vi "OntStatus&Info.vi"(8 "error in":errorcluster caption="错误输入（无错误）", 10 "XML document":string="<?xml version=\"1.0\" encoding=\"utf-8\"?>\n<string xmlns=\"http://CIG_WebService/\"><DOC><Row><CIG_SN>FHTXF4112271</CIG_SN><SSID>ChinaNet-Wrgr</SSID><WAP2>7khcpaes</WAP2><WLP>enguz</WLP><ONT_ID>A013CB-48334A013CB3AC294</ONT_ID><provinceID>HG261GS;unipon_patch_5116_Anhui_CTC_20150609_1645</provinceID><Lot>ZH1509290</Lot><PCBA_Code>13U-00032-21</PCBA_Code><MAC1>A013CB3AC294</MAC1><MAC2>A013CB3AC298</MAC2><Major>NA</Major><Minor>NA</Minor><OEM_SN>FHTTCB3AC294</OEM_SN><BOSA_Code>071-85100-00</BOSA_Code><Hwver>NA</Hwver><MCU>NA</MCU><LoadVer>Anhui20150722.rar/U6</LoadVer><Customer_PN>GPON</Customer_PN></Row></DOC></string>\n\n" caption="XML文档", 11 "XPath expression":string="DOC/Row" caption="XPath表达式") -> (0 "error out":errorcluster caption="错误输出", 3 "OntStatus&Info":string[][](array[string]))   [LabVIEW 2012]
uses:
  <vilib>/xml/Load XML String.vi
  <vilib>/xml/Close Reference(Node).vi
  <vilib>/xml/NI_XML.lvlib
  <resource>/objmgr/DOMUserDefRef.rc
panel:
  out "子字符串":string
  in  "偏移量(0)":i32=39
  out "parse errors":string caption="解析出错"
  out "结果字符串":string
  out "数组":string[](array[string])
  out "match found?":bool caption="找到匹配？"
  out "Result XML":string caption="结果XML"
  # "<?xml version=\"1.0\" encoding=\"utf-8\"?>\n<string xmlns=\"http://CIG_WebService/\">\n<DOC><Row><CIG_SN>081690290863</CIG_SN><CheckResult/><Message/><DuplicatedacQty/><SSID/><WAP2>16a0168b</WAP2><WLP/><ONT_ID/><provinceID/><Lot>ZH1610017</Lot><PCBA_Code>15K-00007-21</PCBA_Code><MAC1/><MAC2/><Major>0090</Major><Minor>23</Minor><OEM_SN>081690290863</OEM_SN><FSAN_SN/><BOSA_Code>071-85200-00</BOSA_Code><Hwver>02</Hwver><MCU>NA</MCU><LoadVer>NA</LoadVer><MFG_Date>2016-10-12</MFG_Date><OEM_PCBA_PN/><SSID1_ID/><SSID2_ID/><SSID2_PWD/><WLanMac1/><WLanMac2/><Customer_PN/><LaserSN/><RFPI/><RFPOWER/><DECT_TYPE/><ServiceTag/><Super_Code>15K-90004</Super_Code><IsHuaWei>N</IsHuaWei><BosaQty>1</BosaQty><ONTIP/></Row></DOC></string>"
  # "<?xml version=\"1.0\" encoding=\"utf-8\"?>\n<string xmlns=\"http://CIG_WebService/\"><?xml version=\"1.0\"?>\n<ROOT>\n<HEAD>\n<RC>SFMS_CE_A1</RC>\n<RCNAME>工装计数</RCNAME>\n<APP_ID>{{2F986A52-32F6-C090-5250-B3035315C7E7}}</APP_ID>\n<AUTH_TOKEN>5K@AANDC@HI_QJbQ\\UT^]b_^uhglpppvl|ll</AUTH_TOKEN>\n<RETURNTYPE></RETURNTYPE>\n<TIMESTAMP>2017-08-16 09:57:13</TIMESTAMP>\n<STATUS>1</STATUS>\n<REMARK></REMARK>\n<LGUID>38407521-9ABA-460F-B7E3-BE3CBE1E5FF6</LGUID>\n<SENDTYPE></SENDTYPE>\n<SENDFROM>MES</SENDFROM>\n</HEAD>\n<SFMS_CE_A1>\n<VIN>AL000131-02</VIN>\n<STATUS>Pop</STATUS>\n<ERRORMSG>AL000131-02还有20次到使用次数，请及时保养！</ERRORMSG>\n</SFMS_CE_A1>\n</ROOT></string>"
  # "<?xml version=\"1.0\" encoding=\"utf-8\"?>\n<string xmlns=\"http://CIG_WebService/\"><?xml version=\"1.0\"?>\n<ROOT>\n<HEAD>\n<RC>MSSF_MTO_A2</RC>\n<RCNAME>工单ATE测试软件信息</RCNAME>\n<APP_ID>{5C128BE7-0FB2-3CCB-4A41-821E960FCCF1}</APP_ID>\n<AUTH_TOKEN>8H8;COTH@E][MJRdfgT]la`^kgh~tsollllz</AUTH_TOKEN>\n<RETURNTYPE></RETURNTYPE>\n<TIMESTAMP>2017-03-15 14:01:22</TIMESTAMP>\n<STATUS>1</STATUS>\n<REMARK>PRD_10000004</REMARK>\n<LGUID>5C128BE7-0FB2-3CCB-4A41-821E960FCCF1</LGUID>\n<SENDTYPE></SENDTYPE>\n<SENDFROM>MES</SENDFROM>\n</HEAD>\n<PTCDETAIL>\n<WO>PRD_10000004</WO>\n<PICID></PICID>\n<LINENO></LINENO>\n<PTCID>_V</PTCID>\n<STATUS></STATUS>\n<CHECKSUM></CHECKSUM>\n<URLLOCATION></URLLOCATION>\n<ATEID>_V</ATEID>\n<VALIDSTART></VALIDSTART>\n<VALIDEND></VALIDEND>\n<REMARK></REMARK>\n<RESULT>Fail</RESULT>\n<ERRORMSG>生产工单PIC未指定！</ERRORMSG>\n</PTCDETAIL>\n</ROOT></string>"
  # "<?xml version=\"1.0\" encoding=\"GB2312\"?>\n<string xmlns=\"http://CIG_WebService/\"><DOC><Row><result>PASS</result><msg/></Row></DOC></Upload_SPCLog_FromAnalysisXMLResult></Upload_SPCLog_FromAnalysisXMLResponse></soap:Body></soap:Envelope>"
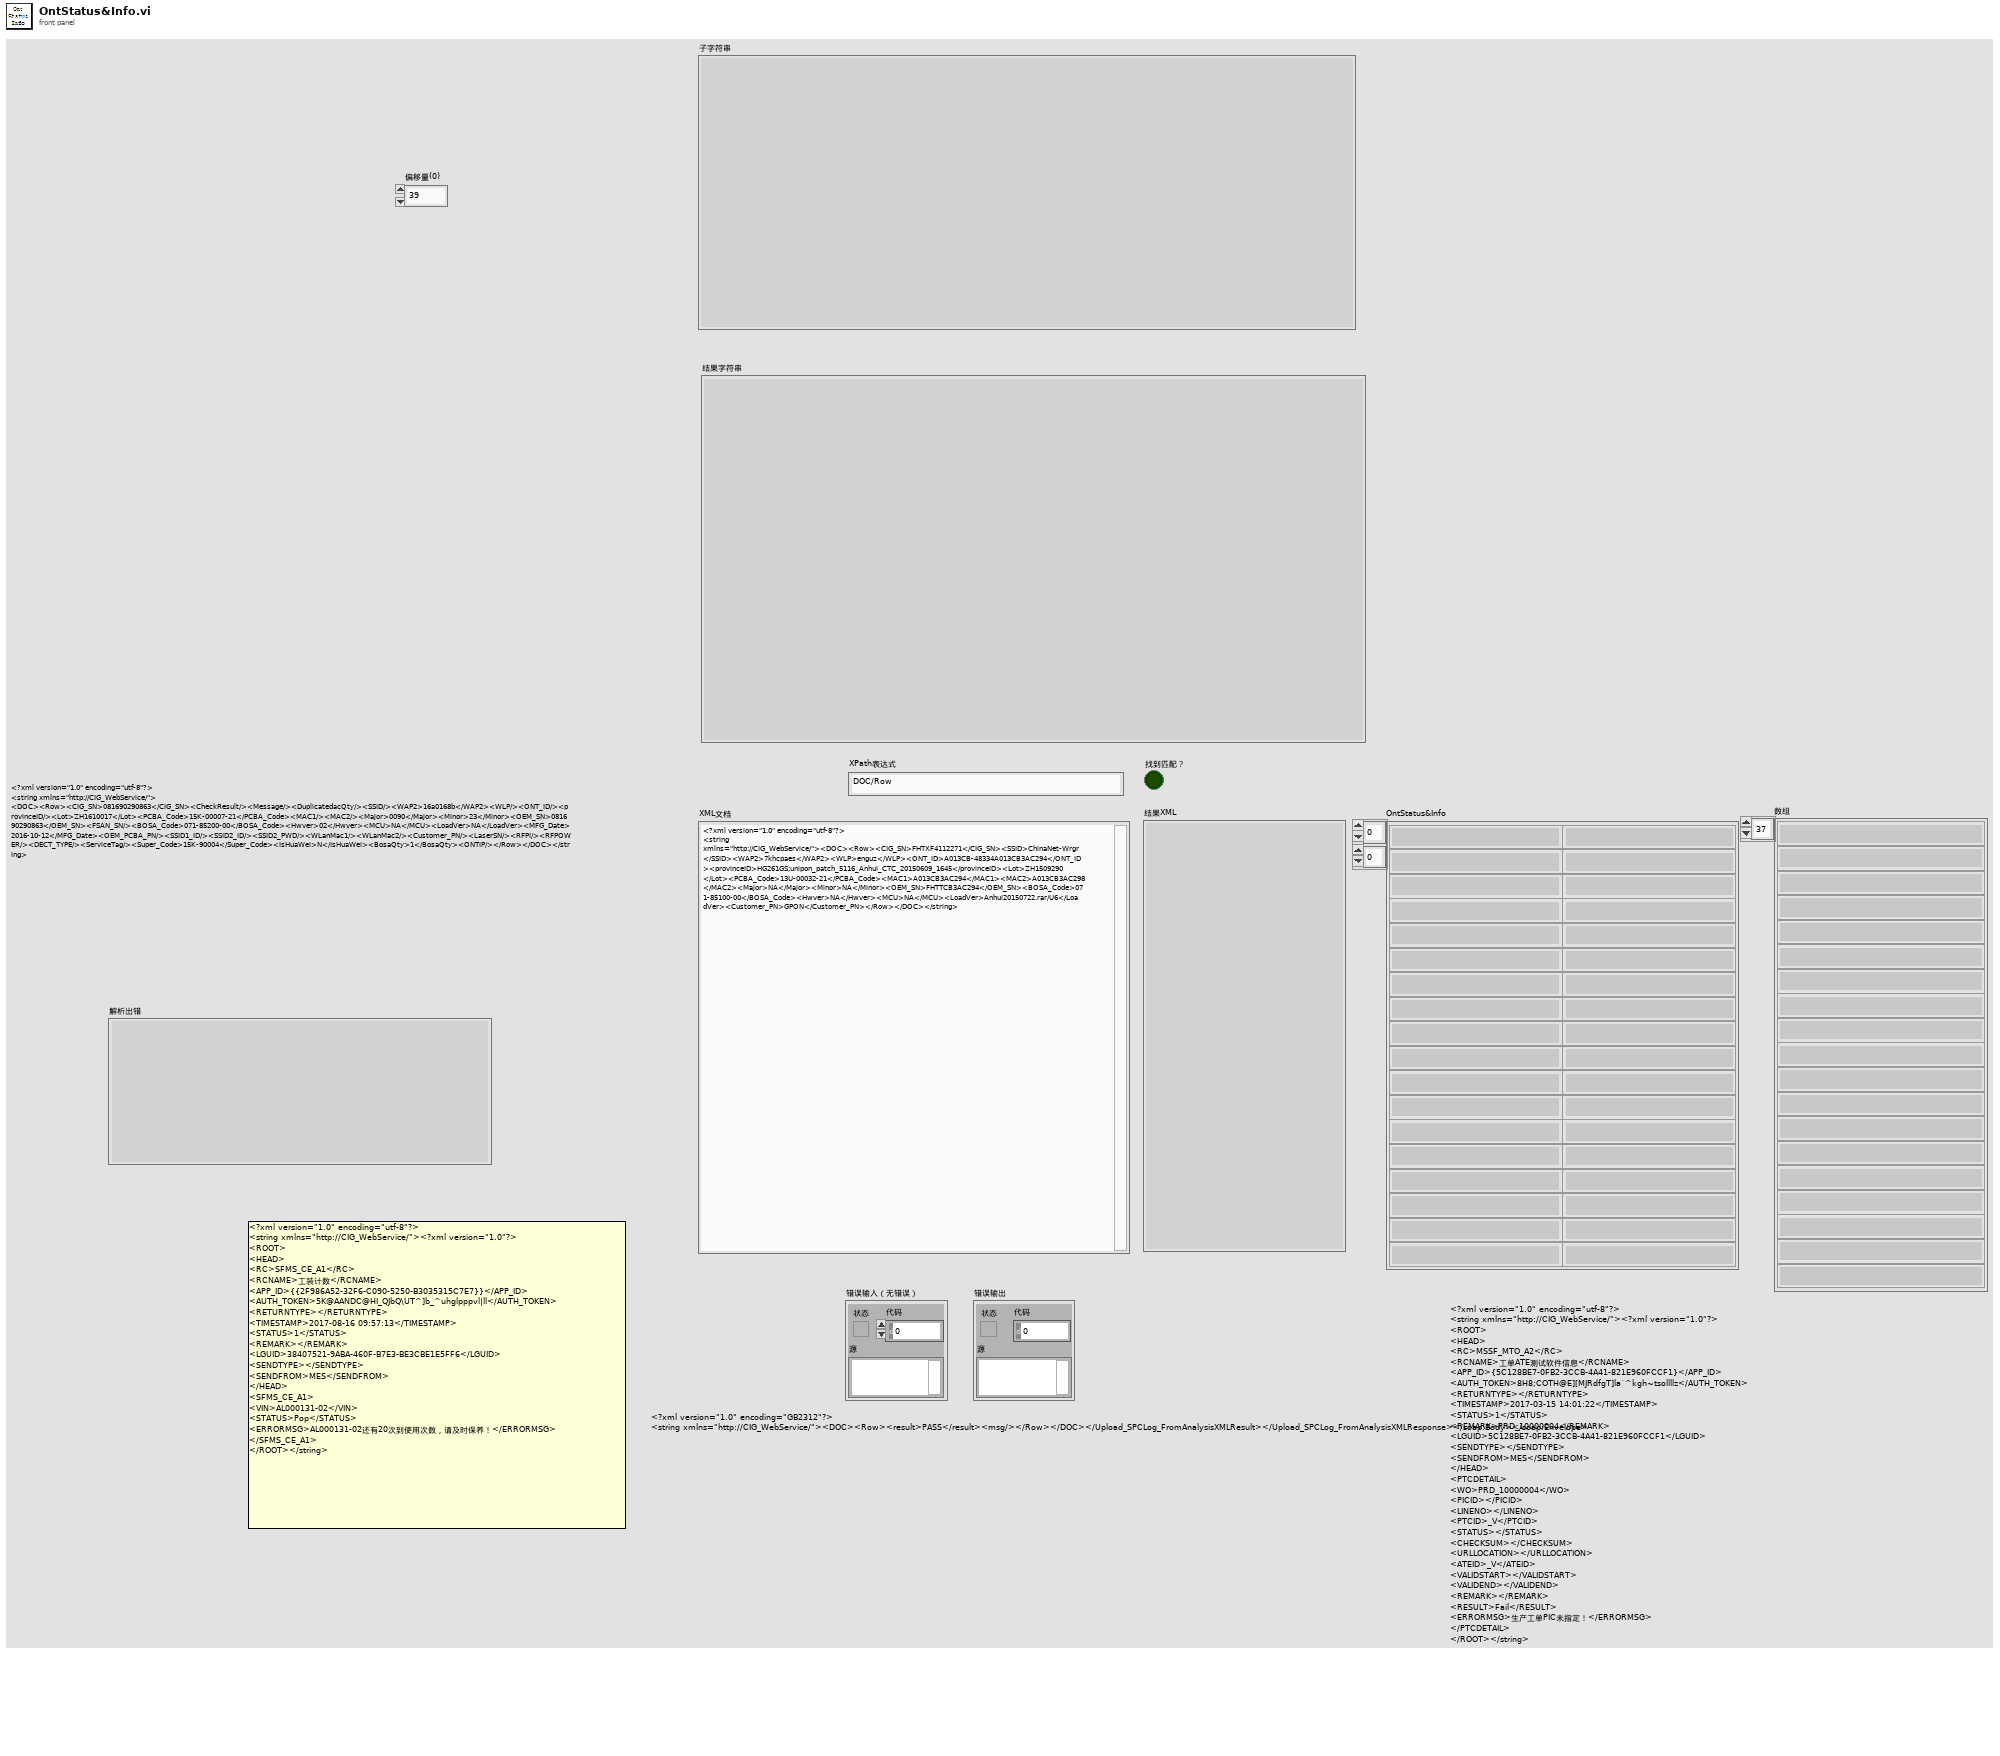
[diagram p1: front panel]
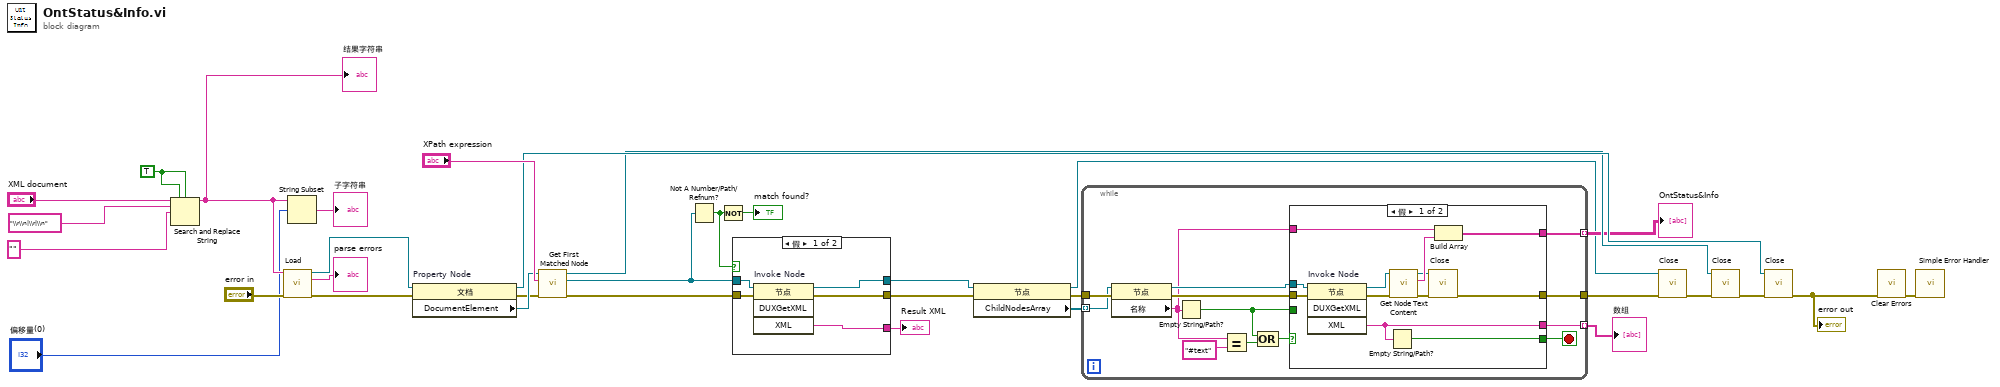
[diagram p0: block diagram]
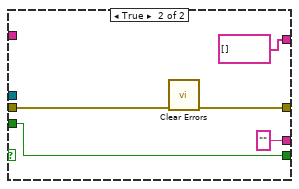
[diagram p2: hidden frame]
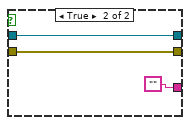
[diagram p3: hidden frame]
diagram:
  w7 = TRUE ("替换全部？(F)")
  n1 = Search and Replace String(replace all?=w7, case sensitive?=w7, input string="XML document", search string="\\r\\n|\\r|\\n" ("搜索字符串"), replace string="" ("替换字符串(\"\")")) -> (result string=w3:string)  [unwired: 3 in, 3 out]
  "结果字符串" <- w3
  n2 = call-poly <vilib>:"Load.vi"("XML string"=w3, "error in (no error)"="error in") -> ("DOM document out"=w31:refnum<k20>, "parse errors"=→"parse errors":string, "error out"=w29:errorcluster)  [unwired: 11 out]
  n3 = String Subset(string=w3, offset (0)="偏移量(0)") -> (substring=→"子字符串":string)  [unwired: 1 in]
  n4 = property on="Property Node" class="文档"(reference=w31, error in=w29) -> (reference out=w26:refnum<k20>, error out=w28:errorcluster, "DocumentElement"=w30:refnum<k20>)
  n5 = call <vilib>:"Get First Matched Node.vi"("error in (no error)"=w28, "XPath expression"="XPath expression", "node in"=w30) -> ("error out"=w20:errorcluster, "node result"=w19:refnum<k20>, "node out"=w21:refnum<k20>)  [unwired: 6 out]
  n6 = Not A Number/Path/Refnum?(number/path/refnum=w19) -> (NaN/Path/Refnum?=w22:bool)
  n7 = Not(x=w22) -> (.not. x?=→"match found?":bool)
  n8 = case shown="假" w22 {
    tunnel: w20 -> [w38 w41]
    tunnel: [w35 w40] -> w17
    tunnel: [w34 w41] -> w16
    tunnel: [w37 ""] -> w24
    tunnel: w19 -> [w36 w40]
    frame False {
      n9 = invoke on="Invoke Node" class="节点" method="DUXGetXML"(reference=w36, error in=w38) -> (reference out=w35:refnum<k20>, error out=w34:errorcluster, "XML"=w37:string)  [unwired: 2 in, 1 out]
    }
    frame True {
    }
  }
  "Result XML" <- w24
  n10 = property on="属性节点" class="节点"(reference=w17, error in=w16) -> (reference out=w11:refnum<k20>, error out=w18:errorcluster, "ChildNodesArray"=w12:refnum<k20>[])
  n11 = while {
    tunnel: [w51] -> w10 mode=indexing
    tunnel: w18 -> [w54]
    tunnel: [w50] -> w14 mode=indexing
    tunnel: [w47] -> w13
    tunnel: w12 -> [w48] mode=indexing
    stop <- w52 stop-if-true
    n12 = property on="属性节点" class="节点"(reference=w48, error in=w54) -> (reference out=w49:refnum<k20>, error out=w53:errorcluster, "名称"=w46:string)
    n13 = Empty String/Path?(string/path=w46) -> (empty?=w42:bool)
    n14 = Equal?(x=w46, y="#text") -> (x = y?=w43:bool)
    n15 = Compound Arithmetic op=OR(w42, w43) -> (w44:bool)
    n16 = case shown="假" w44 {
      tunnel: w53 -> [w66 w71]
      tunnel: [w65 w67] -> w52
      tunnel: [w64 "" ("XML")] -> w51
      tunnel: [w63 string[] []] -> w50
      tunnel: w49 -> [w59 _]
      tunnel: [w57 w70] -> w47
      tunnel: w46 -> [w55 _]
      tunnel: w42 -> [_ w67]
      frame False {
        n17 = invoke on="Invoke Node" class="节点" method="DUXGetXML"(reference=w59, error in=w66) -> (reference out=w62:refnum<k20>, error out=w61:errorcluster, "XML"=w64:string)  [unwired: 2 in, 1 out]
        n18 = Empty String/Path?(string/path=w64) -> (empty?=w65:bool)
        n19 = call <vilib>:"Get Node Text Content.vi"("error in (no error)"=w61, "node in"=w62) -> ("error out"=w58:errorcluster, "node text"=w60:string, "node out"=w56:refnum<k20>)  [unwired: 7 in]
        n20 = call-poly <vilib>:"Close.vi"("error in (no error)"=w58, "node"=w56) -> ("error out"=w57:errorcluster)  [unwired: 7 out]
        n21 = Build Array(w55, w60) -> (w63:string[])
      }
      frame True {
        n22 = call <vilib>:"Clear Errors.vi"("error in (no error)"=w71) -> ("error out"=w70:errorcluster)  [unwired: 6 in]
      }
    }
  }
  "数组" <- w10
  "OntStatus&Info" <- w14
  n23 = call-poly <vilib>:"Close.vi"("error in (no error)"=w13, "node"=w11) -> ("error out"=w32:errorcluster)  [unwired: 7 out]
  n24 = call-poly <vilib>:"Close.vi"("error in (no error)"=w32, "node"=w21) -> ("error out"=w27:errorcluster)  [unwired: 7 out]
  n25 = call-poly <vilib>:"Close.vi"("error in (no error)"=w27, "node"=w26) -> ("error out"=w25:errorcluster)  [unwired: 7 out]
  "error out" <- w25
  n26 = call <vilib>:"Clear Errors.vi"("error in (no error)"=w25) -> ("error out"=w15:errorcluster)  [unwired: 6 in]
  n27 = call <vilib>:"Simple Error Handler.vi"("error in (no error)"=w15) -> ()  [unwired: 1 in, 8 out]
